vi "Connect_CallbackIn_I32.vi"(4 "Slot VI":refnum<vi>, 6 "Receiver":refnum<class "LQObject.lvclass">, 8 "Error In":errorcluster, 10 "Signal":string, 11 "Sender In":refnum<class "LQObject.lvclass">) -> (0 "Error Out":errorcluster, 3 "Sender Out":refnum<class "LQObject.lvclass">)   [LabVIEW 2014, in "LQ Core.lvlib" / "LQCoreEngine.lvclass"]
uses:
  LQCoreEngine.lvclass
  LQObject/LQObject.lvclass
panel:
  # "Copyright (c) 2016 Sze Howe Koh\n\nThis Source Code Form is subject to the terms of the Mozilla Public\nLicense, v. 2.0. If a copy of the MPL was not distributed with this\nfile, You can obtain one at http://mozilla.org/MPL/2.0/."
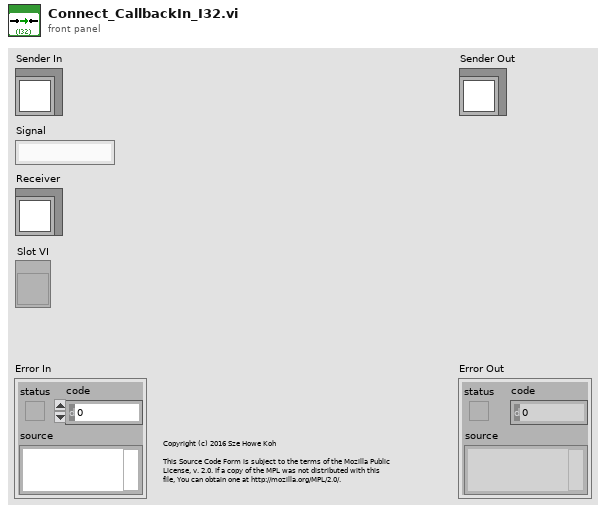
[diagram p1: front panel]
types:
  T1 = cluster{"Receiver":refnum<class "LQObject.lvclass">, "Slot VI":refnum<vi>}
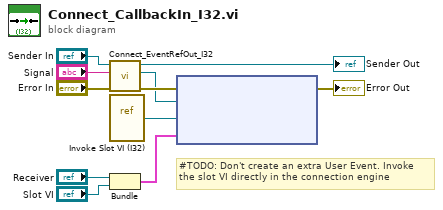
[diagram p0: block diagram]
diagram:
  # "#TODO: Don't create an extra User Event. Invoke\nthe slot VI directly in the connection engine"
  n1 = call "Connect_EventRefOut_I32.vi"("Error In"="Error In", "Signal Signature"="Signal", "Sender In"="Sender In") -> ("Error Out"=w11:errorcluster, "I32 Signal"=w6:refnum<user-event>, "Sender Out"=→"Sender Out":refnum<class "LQObject.lvclass">)  [unwired: 6 in]
  n2 = vi-ref "Invoke Slot VI (I32).vi"() -> ("vi reference"=w1:refnum<vi>)
  n3 = Bundle("Receiver"="Receiver", "Slot VI"="Slot VI") -> (w2:T1)  [unwired: 1 in]
  n4 = node(w11, w6, w1, w2) -> (→"Error Out":errorcluster)  [unwired: 1 in, 1 out]
